vi "Populate Field.vi"(8 "error in (no error)":errorcluster, 10 "Field Name Array (All)":string[](array[string]), 11 "Panel Form Controller in":refnum<class "Panel Form Controller.lvclass">) -> (0 "error out":errorcluster, 3 "Panel Form Controller out":refnum<class "Panel Form Controller.lvclass">)   [LabVIEW 2020, in "Panel Form Controller.lvlib" / "Panel Form Controller.lvclass"]
uses:
  Panel Form Controller.lvclass
  Panel Form Controller.lvclass/Panel Form Controller.ctl
  Database OOP/Table Libraries/Basic Form/Basic Form.lvclass
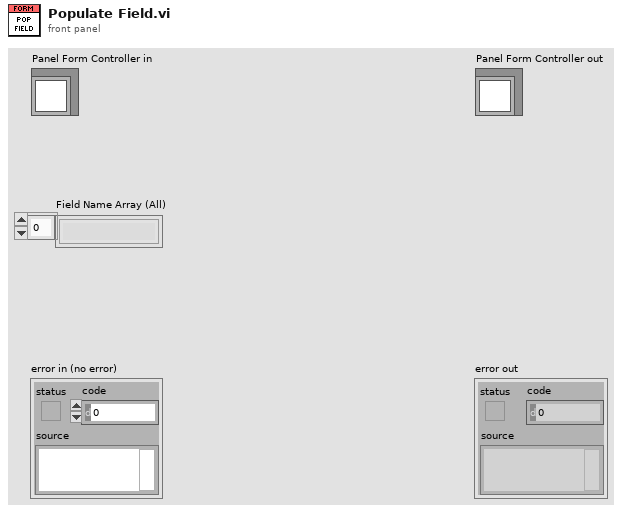
[diagram p1: front panel]
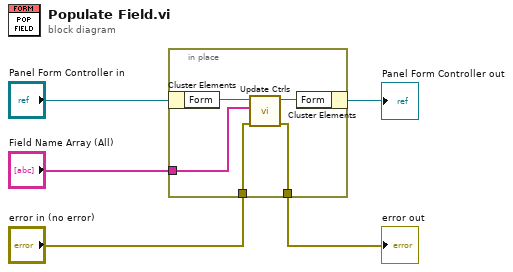
[diagram p0: block diagram]
diagram:
  n1 = in-place {
    in-place-border: "Field Name Array (All)" -> [w8]
    in-place-border: "error in (no error)" -> [w7]
    in-place-border: [w6] -> w2
    n2 = in-place-cluster #1("Panel Form Controller in") -> ("Form"=w10:refnum<class "Basic Form.lvclass">)
    n3 = call "Update Ctrls.vi"("error in (no error)"=w7, "Columns (All)"=w8, "Basic Form in"=w10) -> ("error out"=w6:errorcluster, "Basic Form out"=w9:refnum<class "Basic Form.lvclass">)  [unwired: 7 in]
    n4 = in-place-cluster #1("Form"=w9) -> (→"Panel Form Controller out":refnum<class "Panel Form Controller.lvclass">)
  }
  "error out" <- w2
